vi "DivideByNCounter.vi"(6 "Output Terminal":tag="/Dev1/PFI8", 8 "error in":errorcluster, 9 "Counter":tag="Dev1/ctr7", 10 "Input Terminal":tag="/Dev1/PFI11", 11 "Divide By N":dbl=300000.0 format="%.6f") -> (0 "error out":errorcluster, 3 "task out":refnum<k21>)   [LabVIEW 2014]
doc: "This example demonstrates how to generate a single pulse using a counter output. \n\nThe single pulse may be triggered once or repeatedly from an external source."
uses:
  <vilib>/DAQmx/create/channels.llb/DAQmx Create Channel (CO-Pulse Generation-Ticks).vi
  <vilib>/DAQmx/configure/timing.llb/DAQmx Timing (Implicit).vi
  <resource>/objmgr/daqmx.rc
panel:
  # "Channel Settings"
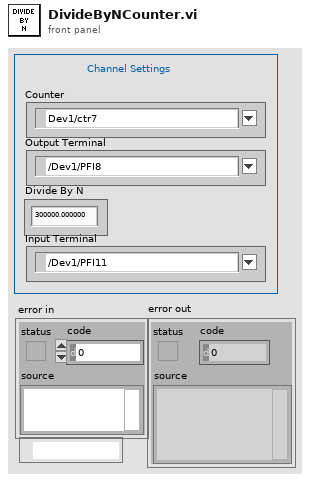
[diagram p1: front panel]
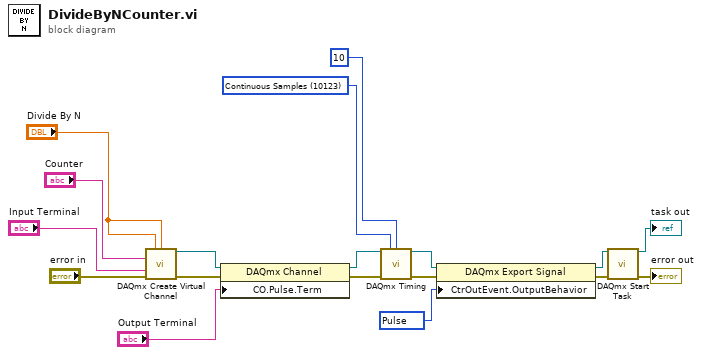
[diagram p0: block diagram]
diagram:
  w11 = 10265 items=["Pulse"=10265, "Toggle"=10307] ("CtrOutEvent.OutputBehavior")
  w13 = 10123 items=["Finite Samples"=10178, "Continuous Samples"=10123, "Hardware Timed Single Point"=12522] ("sample mode")
  n1 = call-poly <vilib>:"DAQmx Create Virtual Channel.vi"("high ticks"="Divide By N", "low ticks"="Divide By N", "counter"="Counter", "source of ticks"="Input Terminal", "error in"="error in") -> ("task out"=w10:refnum<k21>, "error out"=w17:errorcluster)  [unwired: 9 in]
  n2 = property class="DAQmx Channel"(reference=w10, error in=w17, "CO.Pulse.Term"="Output Terminal") -> (reference out=w9:refnum<k21>, error out=w8:errorcluster)
  n3 = call-poly <vilib>:"DAQmx Timing.vi"("task/channels in"=w9, "sample mode"=w13, "samples per channel"=10, "error in"=w8) -> ("task out"=w12:refnum<k21>, "error out"=w7:errorcluster)  [unwired: 10 in]
  n4 = property class="DAQmx Export Signal"(reference=w12, error in=w7, "CtrOutEvent.OutputBehavior"=w11) -> (reference out=w4:refnum<k21>, error out=w3:errorcluster)
  n5 = call <vilib>:"DAQmx Start Task.vi"("task/channels in"=w4, "error in"=w3) -> ("task out"=→"task out":refnum<k21>, "error out"=→"error out":errorcluster)  [unwired: 12 in]
